vi "Execution Unit.Async.vi"(10 "Parameters":variant, 11 "Process":refnum<class "Process.lvclass">) -> ()   [LabVIEW 2020, in "AIM MIL-STD-1553 Engine.lvlib" / "Custom Device.lvlib"]
uses:
  Custom Device.lvlib
  <vilib>/NI/NIVS Inline Async API/_VS Inline Async API/Process/Process.lvclass
  <vilib>/NI/NIVS Inline Async API/_Data Access Engine/Data Access Engine/Data Access Engine.lvclass
  Asynchronous Execution Unit Runtime Information.ctl
  Interfaces/Execution Unit/Execution Unit.lvclass
  Interfaces/Shared Resources/Shared Resources.lvclass
  Asynchronous Process Parameters.ctl
  <vilib>/NI/NIVS Inline Async API/_Data Access Engine/Access Type Classes/ReadWrite/ReadWrite.lvclass
  <vilib>/NI/NIVS Inline Async API/_Data Access Engine/Data Access Engine/Methods/ReadWrite.Data.vi
  <vilib>/NI/NIVS Inline Async API/_Data Access Engine/Data Access Engine/Methods/ReadWrite.Data.Reset.vi
  <vilib>/NI/NIVS Inline Async API/_Data Access Engine/Data Access Engine/Methods/Read.Data.vi
  <vilib>/NI/NIVS Inline Async API/_Data Access Engine/Data Access Engine/Methods/ReadWrite.Lookup.vi
  <vilib>/NI/NIVS Inline Async API/_Data Access Engine/Data Access Engine/Methods/Read.Lookup.vi
  <vilib>/NI/NIVS Inline Async API/_Data Access Engine/Data Access Engine/Methods/Write.Lookup.vi
  <vilib>/NI/NIVS Inline Async API/_Data Access Engine/Data Access Engine/Methods/Write.Data.vi
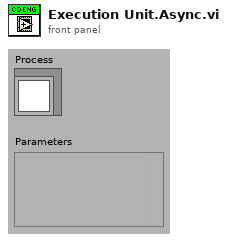
[diagram p1: front panel]
types:
  T1 = typedef "AIM MIL-STD-1553 Engine.lvlib/Custom Device.lvlib/Asynchronous Process Parameters.ctl" = cluster{"Grouped Asynchronous Execution Unit Runtime Information":T2[], "shared resources":refnum<class "Shared Resources.lvclass">}
  T2 = typedef "AIM MIL-STD-1553 Engine.lvlib/Custom Device.lvlib/Asynchronous Execution Unit Runtime Information.ctl" = cluster{"Execution Unit":refnum<class "Execution Unit.lvclass">, "Incoming Channel Group Name":string, "Outgoing Channel Group Name":string, "ReadWrite Channel Group Name":string}
  T3 = typedef "Data Access Engine.lvlib/Data Access Engine.lvclass/Write.DVR.ctl" = refnum<data-value>
  T4 = typedef "Data Access Engine.lvlib/Data Access Engine.lvclass/ReadWrite.DVR.ctl" = refnum<data-value>
  T5 = typedef "Data Access Engine.lvlib/Data Access Engine.lvclass/Read.DVR.ctl" = refnum<data-value>
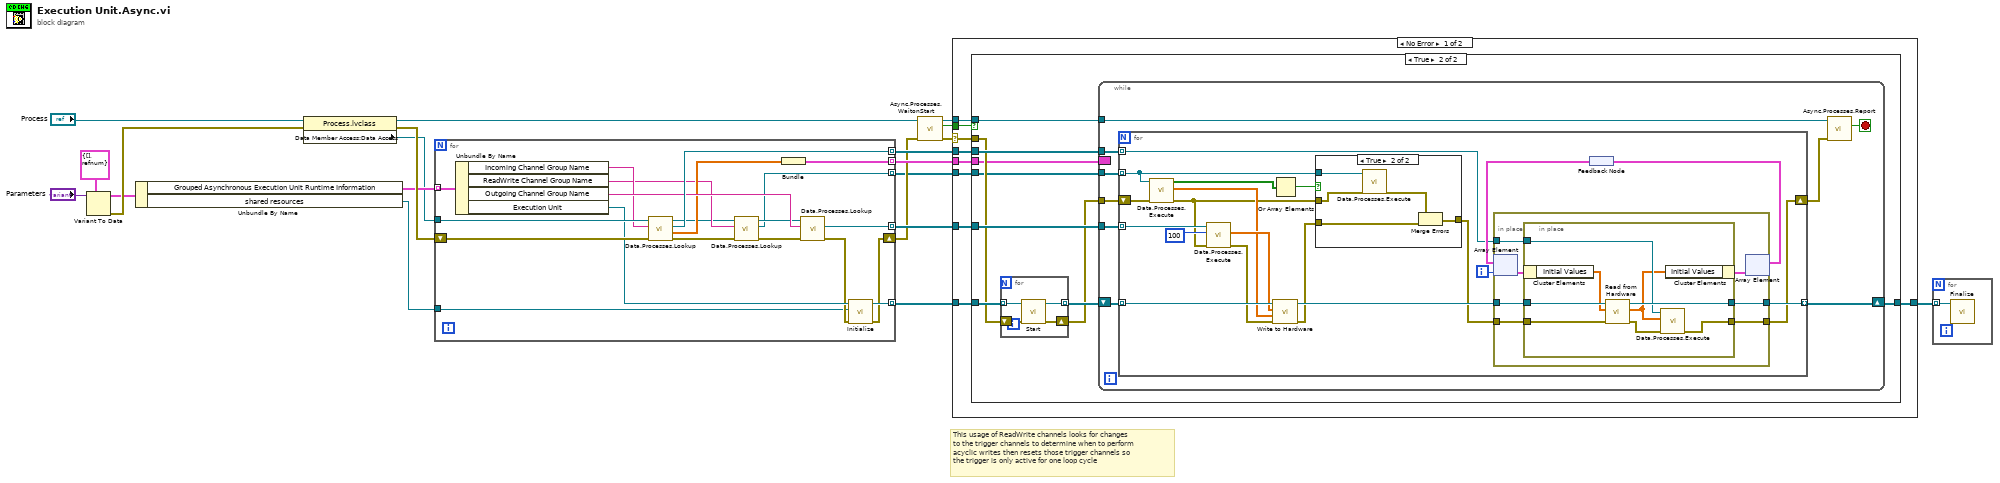
[diagram p0: block diagram]
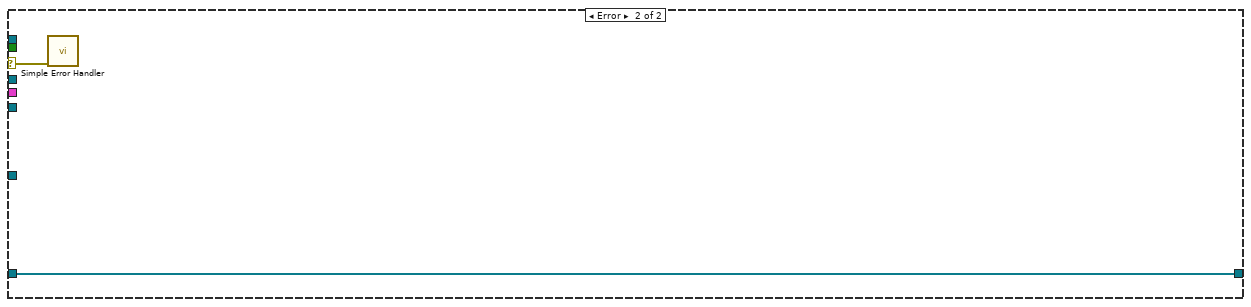
[diagram p4: hidden frame]
diagram:
  # "This usage of ReadWrite channels looks for changes\nto the trigger channels to determine when to perform\nacyclic writes then resets those trigger channels so\nthe trigger is only active for one loop cycle"
  n1 = Variant To Data(type=T1 {"Grouped Asynchronous Execution Unit Runtime Information"=[], "shared resources"=refnum} ("Asynchronous Process Parameters"), Variant="Parameters") -> (data=w9:T1, error out=w10:errorcluster)  [unwired: 1 in]
  n2 = Unbundle By Name(w9) -> ("Grouped Asynchronous Execution Unit Runtime Information"=w3:T2[], "shared resources"=w1:refnum<class "Shared Resources.lvclass">)
  n3 = property class="Process.lvclass"(reference="Process", error in=w10) -> (reference out=w14:refnum<class "Process.lvclass">, error out=w13:errorcluster, "Data Member Access:Data Access"=w2:refnum<class "Data Access Engine.lvclass">)
  n4 = for {
    tunnel: [w40] -> w17 mode=indexing
    tunnel: [w39] -> w16 mode=indexing
    tunnel: w2 -> [w38]
    tunnel: [w22] -> w8 mode=indexing
    tunnel: [w33] -> w7 mode=indexing
    tunnel: [w26] -> w4 mode=indexing
    tunnel: w3 -> [w23] mode=indexing
    shift-right: [w31] -> w6
    shift-left: w13 -> [w37]
    tunnel: w1 -> [w21]
    n5 = Unbundle By Name(w23) -> ("Incoming Channel Group Name"=w30:string, "ReadWrite Channel Group Name"=w29:string, "Outgoing Channel Group Name"=w36:string, "Execution Unit"=w34:refnum<class "Execution Unit.lvclass">)
    n6 = call-poly <vilib>:"Data.Processes.Lookup.vi"("error in (no error)"=w37, "Name"=w30, "Data Access API in"=w38) -> ("error out"=w25:errorcluster, "Initial Values"=w35:dbl[], "Ref"=w39:T3, "Data Access API out"=w28:refnum<class "Data Access Engine.lvclass">)  [unwired: 5 in]
    n7 = call-poly <vilib>:"Data.Processes.Lookup.vi"("error in (no error)"=w25, "Name"=w29, "Data Access API in"=w28) -> ("error out"=w24:errorcluster, "Ref"=w26:T4, "Data Access API out"=w27:refnum<class "Data Access Engine.lvclass">)  [unwired: 5 in, 1 out]
    n8 = Bundle("Initial Values"=w35) -> (w22:cluster{"Initial Values":dbl[]})  [unwired: 1 in]
    n9 = call-poly <vilib>:"Data.Processes.Lookup.vi"("error in (no error)"=w24, "Name"=w36, "Data Access API in"=w27) -> ("error out"=w32:errorcluster, "Ref"=w40:T5)  [unwired: 5 in, 2 out]
    n10 = call-dynamic "Initialize.vi"("error in (no error)"=w32, "shared resources"=w21, "Execution Unit in"=w34) -> ("error out"=w31:errorcluster, "Execution Unit out"=w33:refnum<class "Execution Unit.lvclass">)  [unwired: 7 in]
  }
  n11 = call <vilib>:"Async.Processes.WaitonStart.vi"("error in (no error)"=w6, "Process"=w14) -> ("error out"=w18:errorcluster, "Execute"=w20:bool, "Process out"=w19:refnum<class "Process.lvclass">)  [unwired: 7 in]
  n12 = case shown="No Error" w18 {
    selector: w18 -> [w45 w116]
    tunnel: w20 -> [w49 _]
    tunnel: w19 -> [w48 _]
    tunnel: w16 -> [w47 _]
    tunnel: w17 -> [w46 _]
    tunnel: w8 -> [w44 _]
    tunnel: w7 -> [w43 w115]
    tunnel: [w42 w115] -> w5
    tunnel: w4 -> [w41 _]
    frame No Error {
      n13 = case shown="True" w49 {
        tunnel: w45 -> [_ w56]
        tunnel: w48 -> [_ w58]
        tunnel: w46 -> [_ w60]
        tunnel: w47 -> [_ w59]
        tunnel: w44 -> [_ w54]
        tunnel: w43 -> [w50 w57]
        tunnel: [w50 w53] -> w42
        tunnel: w41 -> [_ w52]
        frame False {
        }
        frame True {
          n14 = for {
            shift-right: [w61] -> w51
            shift-left: w56 -> [w63]
            tunnel: w57 -> [w64] mode=indexing
            tunnel: [w62] -> w55 mode=indexing
            n15 = call-dynamic "Start.vi"("error in (no error)"=w63, "Execution Unit in"=w64) -> ("error out"=w61:errorcluster, "Execution Unit out"=w62:refnum<class "Execution Unit.lvclass">)  [unwired: 8 in]
          }
          n16 = while {
            tunnel: w58 -> [w73]
            tunnel: w60 -> [w71]
            tunnel: w59 -> [w70]
            border: w54 -> [_]
            shift-right: [w68] -> w53
            shift-left: w55 -> [w69]
            tunnel: w52 -> [w67]
            tunnel: w51 -> [w66]
            stop <- w72 stop-if-true
            n17 = for {
              tunnel: w71 -> [w93] mode=indexing
              tunnel: w70 -> [w74] mode=indexing
              tunnel: w69 -> [w91] mode=indexing
              tunnel: [w87] -> w68 mode=indexing
              tunnel: w67 -> [w86] mode=indexing
              shift-right: [w75] -> w65
              shift-left: w66 -> [w85]
              i -> [w78]
              n18 = call-poly <vilib>:"Data.Processes.Execute.vi"("error in (no error)"=w85, "Ref"=w86) -> ("error out"=w81:errorcluster, "Data"=w84:dbl[], "Detect?"=w83:bool[])  [unwired: 6 in, 1 out]
              n19 = call-poly <vilib>:"Data.Processes.Execute.vi"("error in (no error)"=w81, "timeout ms"=100, "Ref"=w93) -> ("error out"=w88:errorcluster, "Values"=w89:dbl[])  [unwired: 6 in, 1 out]
              n20 = call-dynamic "Write to Hardware.vi"("error in (no error)"=w88, "Trigger Values"=w84, "Values in"=w89, "Execution Unit in"=w91) -> ("error out"=w80:errorcluster, "Execution Unit out"=w90:refnum<class "Execution Unit.lvclass">)  [unwired: 4 in, 2 out]
              n21 = Or Array Elements(Boolean array=w83) -> (logical OR=w82:bool)
              n22 = case shown="True" w82 {
                tunnel: w86 -> [_ w114]
                tunnel: w81 -> [_ w112]
                tunnel: w80 -> [w109 w113]
                tunnel: [w109 w110] -> w79
                frame False {
                }
                frame True {
                  n23 = call-poly <vilib>:"Data.Processes.Execute.vi"("error in (no error)"=w112, "Ref"=w114) -> ("error out"=w111:errorcluster)  [unwired: 8 in, 1 out]
                  n24 = Merge Errors(w111, w113) -> (w110:errorcluster)
                }
              }
              n25 = feedback #1() -> (w77:cluster{"Initial Values":dbl[]}[])
              n26 = in-place {
                in-place-border: w90 -> [w100]
                in-place-border: [w99] -> w75
                in-place-border: [w98] -> w87
                in-place-border: w79 -> [w97]
                in-place-border: w74 -> [w94]
                n27 = in-place-array #2(w77, w78) -> (w96:cluster{"Initial Values":dbl[]})
                n28 = in-place {
                  in-place-border: w100 -> [w108]
                  in-place-border: [w103] -> w99
                  in-place-border: [w107] -> w98
                  in-place-border: w97 -> [w106]
                  in-place-border: w94 -> [w102]
                  n29 = in-place-cluster #3(w96) -> ("Initial Values"=w105:dbl[])
                  n30 = call-dynamic "Read from Hardware.vi"("error in (no error)"=w106, "Values in"=w105, "Execution Unit in"=w108) -> ("error out"=w104:errorcluster, "Values out"=w101:dbl[], "Execution Unit out"=w107:refnum<class "Execution Unit.lvclass">)  [unwired: 6 in]
                  n31 = call-poly <vilib>:"Data.Processes.Execute.vi"("error in (no error)"=w104, "Values"=w101, "Ref"=w102) -> ("error out"=w103:errorcluster)  [unwired: 8 in]
                  n32 = in-place-cluster #3("Initial Values"=w101) -> (w95:cluster{"Initial Values":dbl[]})
                }
                n33 = in-place-array #2(w95) -> (w76:cluster{"Initial Values":dbl[]}[])  [unwired: 1 out]
              }
              n34 = feedback-in #1(w76) -> ()
            }
            n35 = call <vilib>:"Async.Processes.Report.vi"("Error"=w65, "Process in"=w73) -> ("Stop"=w72:bool)  [unwired: 8 in, 1 out]
          }
        }
      }
    }
    frame Error {
      n36 = call <vilib>:"Simple Error Handler.vi"("error in (no error)"=w116) -> ()  [unwired: 4 in, 5 out]
    }
  }
  n37 = for {
    tunnel: w5 -> [w117] mode=indexing
    n38 = call-dynamic "Finalize.vi"("Execution Unit in"=w117) -> ()  [unwired: 9 in, 2 out]
  }
